vi "matlab_base_vi.vi"() -> ()   [LabVIEW 2013]
uses:
  <vilib>/Analysis/2dsp.llb/1D Convolution (CDB).vi
  <vilib>/Analysis/2dsp.llb/Upsample (CDB).vi
  <vilib>/imath/engines/lvmath2/RunTimeEngine/ErrorHandling/NIMS_Finalize Error.vi
  <vilib>/imath/engines/lvmath2/RunTimeEngine/NodeEndStatement/NIMS_NodeEndStatement_Output.vi
  <instcachedir>/0/NIMS_NodeEndStatement_Output_53EC0D466D134D7ABD903AC30B43404B.lvgen/NIMS_NodeEndStatement_Output_53EC0D466D134D7ABD903AC30B43404B_004.vi
  <vilib>/imath/engines/lvmath2/RunTimeEngine/BuiltInFunctions/randint/NIMS_randint(1,I32,RV).vi
  <vilib>/imath/engines/lvmath2/RunTimeEngine/ErrorHandling/NIMS_Create Error From Enums.vi
  <vilib>/Analysis/NI_AALPro.lvlib
panel:
  in  "file (use dialog) 2":path
  in  "file (use dialog)":path
  in  "Sampling frequency 2":dbl=30000000.0
  in  "Sampling frequency":dbl=30000000.0
  out "number of symbols (per block)":dbl
  out "After Matched Filtering":dbl[](graph)
  in  "Symbol frequency 2":dbl
  out "Baseband Signal":dbl[](graph)
  out "Root Raise Cosine Pulse":dbl[](graph)
  out "Constellation (16-QAM)":cdb[](graph)
  in  "Symbol frequency":dbl
  in  "number of bits (per block)":dbl
  # "TX"
  # "Rx"
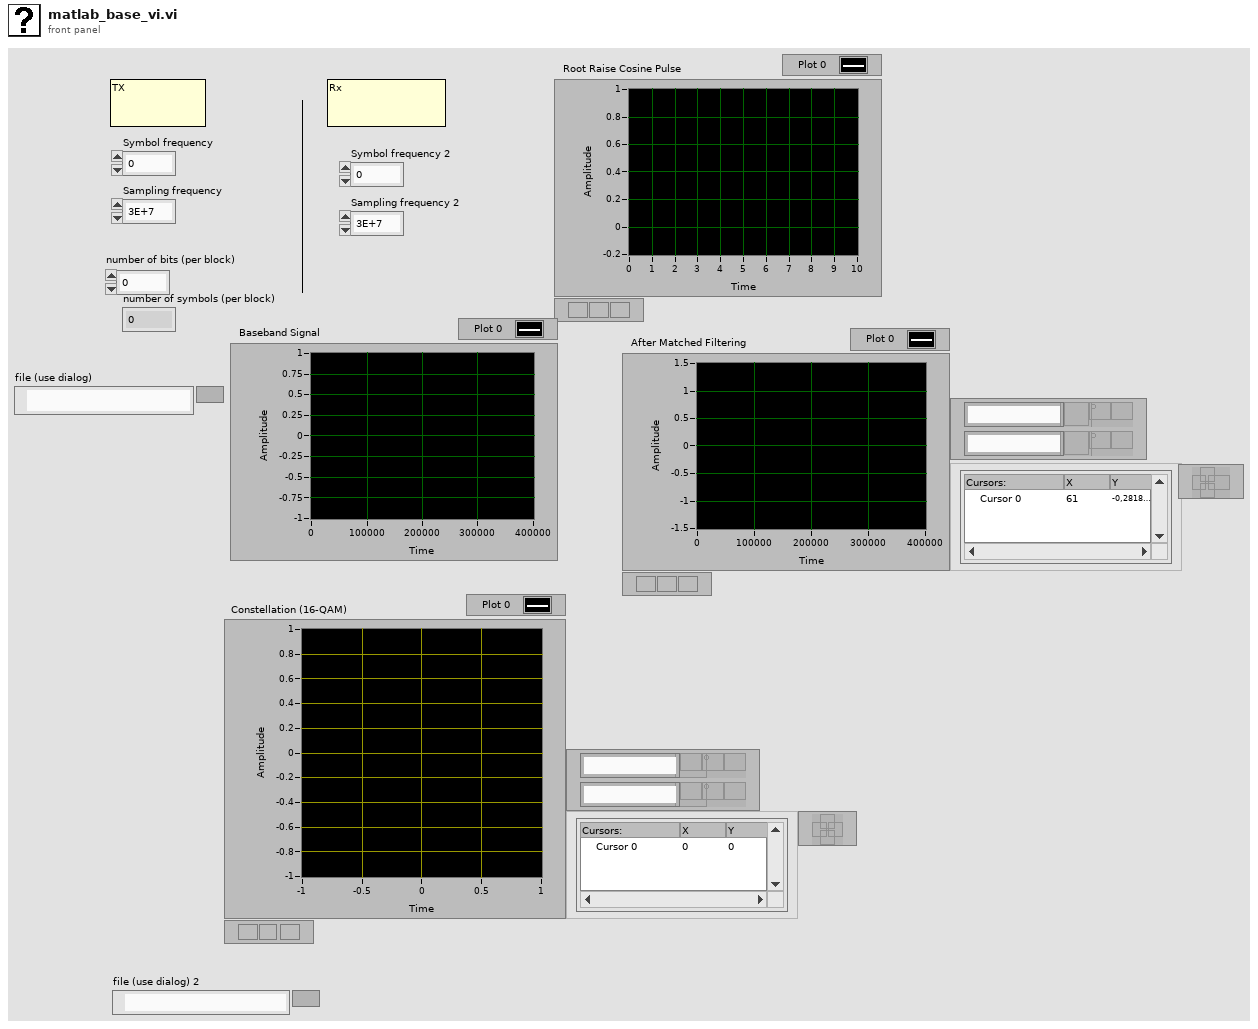
[diagram p1: front panel]
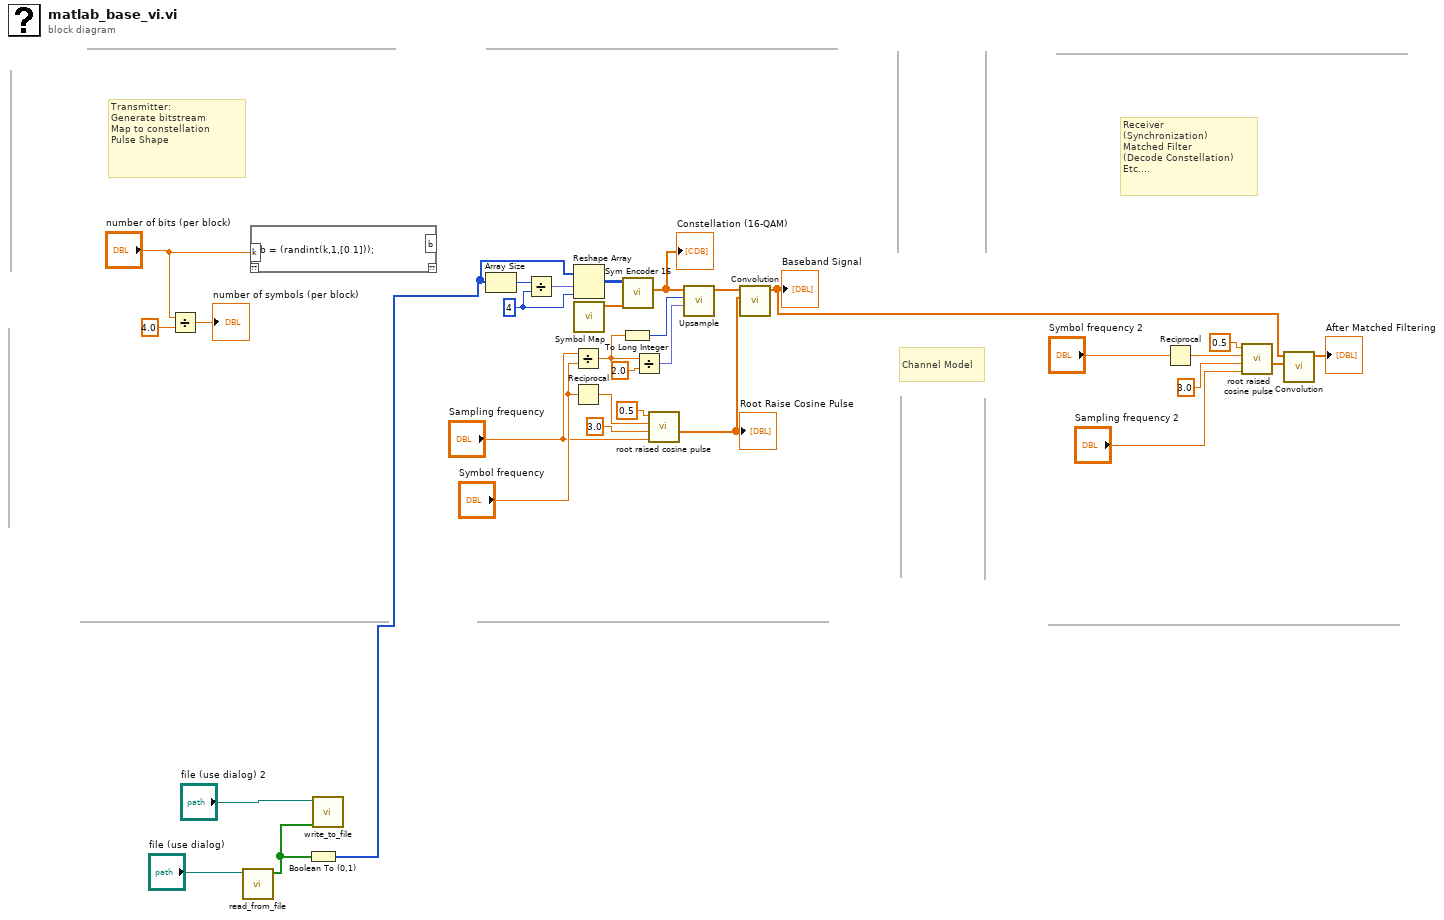
[diagram p0: block diagram]
diagram:
  w28 = 4 ("dimension size")
  # "Channel Model"
  # "Transmitter:\nGenerate bitstream\nMap to constellation\nPulse Shape"
  # "Receiver\n(Synchronization)\nMatched Filter\n(Decode Constellation)\nEtc...."
  n1 = Divide(x="number of bits (per block)", y=4.0) -> (x/y=→"number of symbols (per block)":dbl)
  n2 = call "read_from_file.vi"("file (use dialog)"="file (use dialog)") -> ("data"=w2:bool[])  [unwired: 10 in]
  n3 = mathscript code="b = (randint(k,1,[0 1]));"("k"="number of bits (per block)") -> ()  [unwired: 1 in, 2 out]
  n4 = Boolean To (0,1)(Boolean=w2) -> (0, 1=w1:i16[])
  n5 = call "write_to_file.vi"("data 3"=w2, "file (use dialog) in"="file (use dialog) 2") -> ()  [unwired: 10 in]
  n6 = Array Size(array=w1) -> (size(s)=w30:i32)
  n7 = Divide(x=w30, y=w28) -> (x/y=w29:fxp<+,27,27>)
  n8 = Divide(x="Sampling frequency", y="Symbol frequency") -> (x/y=w21:dbl)
  n9 = Reciprocal(x="Symbol frequency") -> (1/x=w13:dbl)
  n10 = Reshape Array(w1, w29, w28) -> (w26:i16[][])
  n11 = call "Symbol Map.vi"() -> ("symbol_map"=w27:cdb[])  [unwired: 11 in]
  n12 = To Long Integer(number=w21) -> (32bit integer=w20:i32)
  n13 = call "Sym Encoder 16.vi"("symbol_map"=w27, "b"=w26) -> ("a"=w25:cdb[])  [unwired: 9 in]
  "Constellation (16-QAM)" <- w25
  n14 = Divide(x=w21, y=2.0) -> (x/y=w5:fxp<+,32,32>)
  n15 = call "root raised cosine pulse.vi"("fs"="Sampling frequency", "span"=3.0, "tau"=w13, "a"=0.5) -> ("y"=w23:cdb[])  [unwired: 6 in, 1 out]
  "Root Raise Cosine Pulse" <- w23
  n16 = call-poly <vilib>:"Upsample.vi"("leading zeros"=w5, "upsampling factor"=w20, "X"=w25) -> ("Upsampled Array"=w24:cdb[])  [unwired: 7 in, 1 out]
  n17 = call-poly <vilib>:"Convolution.vi"("Y"=w23, "X"=w24) -> ("X * Y"=w16:cdb[])  [unwired: 8 in, 1 out]
  "Baseband Signal" <- w16
  n18 = Reciprocal(x="Symbol frequency 2") -> (1/x=w11:dbl)
  n19 = call "root raised cosine pulse.vi"("fs"="Sampling frequency 2", "span"=3.0, "tau"=w11, "a"=0.5) -> ("y"=w17:cdb[])  [unwired: 6 in, 1 out]
  n20 = call-poly <vilib>:"Convolution.vi"("Y"=w17, "X"=w16) -> ("X * Y"=→"After Matched Filtering":cdb[])  [unwired: 8 in, 1 out]
